vi "Calc Frequencies.vi"(7 "Freq. Type":T1, 8 "error in (no error)":errorcluster, 11 "RPM":dbl) -> (0 "error out":errorcluster, 3 "f":dbl)   [LabVIEW 2026, in "Acquisition.lvlib"]
uses:
  Acquisition.lvlib
  Controls/Frequency Type.ctl
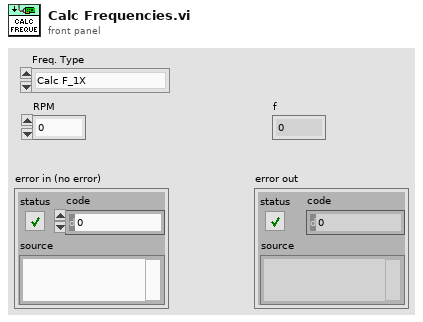
[diagram p1: front panel]
types:
  T1 = typedef "Acquisition.lvlib/Frequency Type.ctl" = enum16{"Calc F_1X", "Calc F_cutoff"}
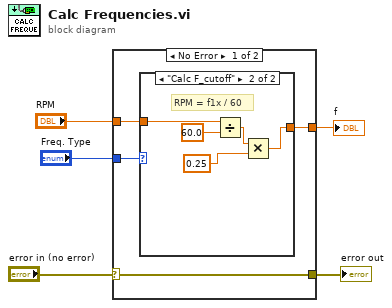
[diagram p0: block diagram]
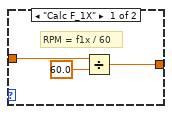
[diagram p2: hidden frame]
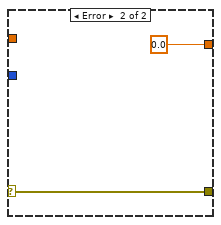
[diagram p3: hidden frame]
diagram:
  n1 = case shown="No Error" "error in (no error)" {
    selector: "error in (no error)" -> [w9 w19]
    tunnel: [w9 w19] -> w4
    tunnel: "RPM" -> [w8 _]
    tunnel: [w7 0.0] -> w2
    tunnel: "Freq. Type" -> [w6 _]
    frame No Error {
      n2 = case shown="\"Calc F_cutoff\"" w6 {
        tunnel: w8 -> [w12 w17]
        tunnel: [w10 w14] -> w7
        frame "Calc F_1X" {
          # "RPM = f1x / 60"
          n3 = Divide(x=w12, y=60.0) -> (x/y=w10:dbl)
        }
        frame "Calc F_cutoff" {
          # "RPM = f1x / 60"
          n4 = Divide(x=w17, y=60.0) -> (x/y=w15:dbl)
          n5 = Multiply(x=w15, y=0.25) -> (x*y=w14:dbl)
        }
      }
    }
    frame Error {
    }
  }
  "error out" <- w4
  "f" <- w2
